vi "OPC UA Server.vi"() -> ()   [LabVIEW 2023]
uses:
  <vilib>/OPCUA/controls/NodeId.ctl
  <vilib>/OPCUA/controls/Data Type.ctl
  <vilib>/OPCUA/NI OPC UA Server.lvlib
panel:
  out "item node ID":T1
  in  "stop":bool
  out "server endpoint URL":string
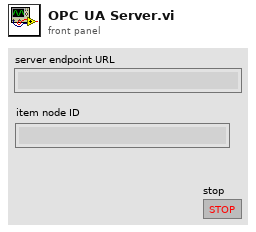
[diagram p1: front panel]
types:
  T1 = typedef "NodeId.ctl" = string
  T2 = typedef "Data Type.ctl" = u16
  T3 = cluster{"name":string, "data type":T2, "access level":u16, "description":string}
  T4 = typedef "OPC UA Server Refnum.ctl" = refnum<k21>
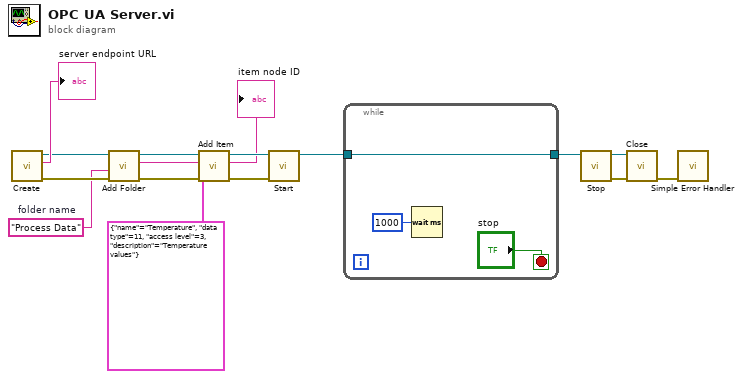
[diagram p0: block diagram]
diagram:
  w4 = "Process Data"  # folder name
  n1 = call <vilib>:"Create.vi"() -> ("error out"=w15:errorcluster, "server endpoint URL"=→"server endpoint URL":string, "OPC UA server refnum out"=w9:T4)  [unwired: 9 in]
  n2 = call <vilib>:"Add Folder.vi"("error in (no error)"=w15, "folder name"=w4, "OPC UA server refnum in"=w9) -> ("error out"=w14:errorcluster, "folder node ID"=w3:T1, "OPC UA server refnum out"=w8:T4)  [unwired: 5 in]
  n3 = call <vilib>:"Add Item.vi"("error in (no error)"=w14, "item"=T3 {"name"="Temperature", "data type"=11, "access level"=3, "description"="Temperature values"}, "parent folder node ID"=w3, "OPC UA server refnum in"=w8) -> ("error out"=w13:errorcluster, "item node ID"=→"item node ID":T1, "OPC UA server refnum out"=w7:T4)  [unwired: 3 in, 1 out]
  n4 = call <vilib>:"Start.vi"("error in (no error)"=w13, "OPC UA server refnum in"=w7) -> ("OPC UA server refnum out"=w6:T4)  [unwired: 7 in, 2 out]
  n5 = while {
    tunnel: w6 -> [w17]
    tunnel: [w17] -> w5
    stop <- "stop" stop-if-true
    n6 = Wait (ms)(milliseconds to wait=u32 1000) -> ()  [unwired: 1 out]
  }
  n7 = call <vilib>:"Stop.vi"("OPC UA server refnum in"=w5) -> ("error out"=w12:errorcluster, "OPC UA server refnum out"=w11:T4)  [unwired: 9 in]
  n8 = call <vilib>:"Close.vi"("error in (no error)"=w12, "OPC UA server refnum in"=w11) -> ("error out"=w10:errorcluster)  [unwired: 9 in]
  n9 = call <vilib>:"Simple Error Handler.vi"("error in (no error)"=w10) -> ()  [unwired: 4 in, 5 out]
